vi "HStest.vi"() -> ()   [LabVIEW 2018]
uses:
  LibTiePie.lvlib
panel:
  out "Stopped?":bool
  in  "ChannelCluster":T1 {"Range" items=["0.2 Vpp"=0.2, "0.4 Vpp"=0.4, "0.8 Vpp"=0.8, "2 Vpp"=2.0, "4 Vpp"=4.0, "8 Vpp"=8.0, "20 Vpp"=20.0, "80 Vpp"=80.0]}
  out "Actual settings":T2
  in  "Settings cluster":T3={"u64RecordLength"=10000, "dPreSampleRatio"=0.2, "dSampleFrequency"=1000000.0, "MeasureMode"=2, "Bitness"=14} {"MeasureMode" items=["Block"=2, "Stream"=1]; "Bitness" items=["16 bit"=16, "14 bit"=14, "12 bit"=12]}
  out "Oscilloscoper cluster":T4
  out "Waveform Chart":dbl[][](graph)
  out "Data Out":dbl[][](array[numeric])
  out "Channel info":T5
  out "Error out":errorcluster
  out "ID out":u32
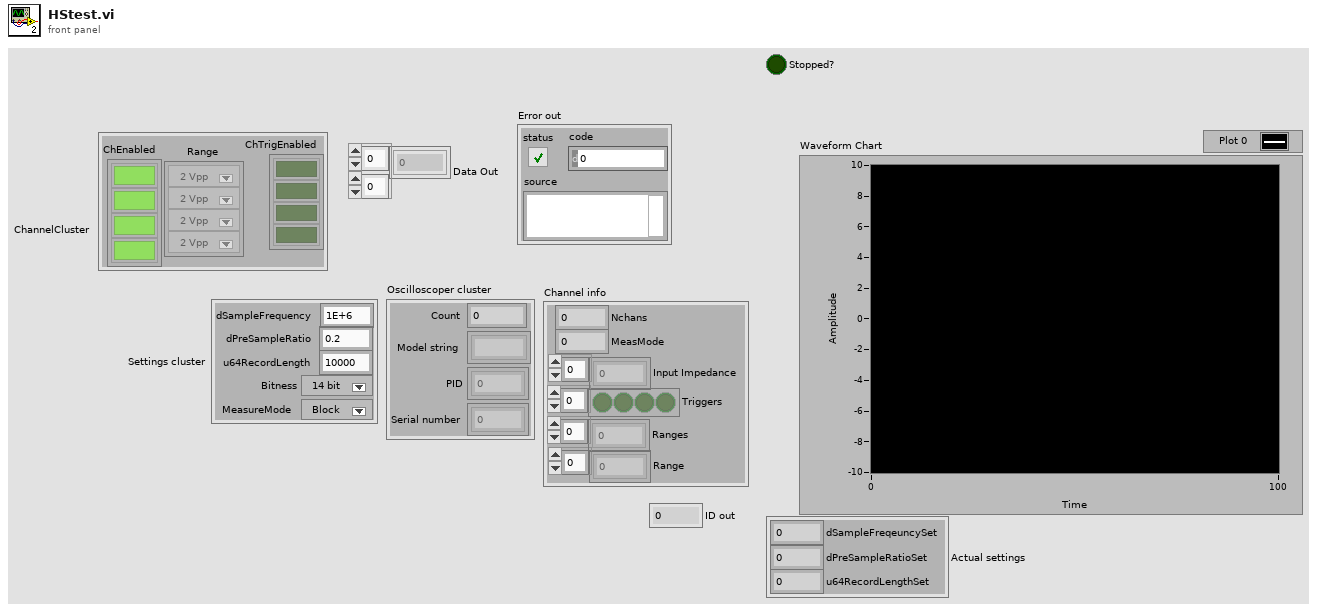
[diagram p1: front panel]
types:
  T1 = cluster{"ChEnabled":bool[], "Range":dbl[], "ChTrigEnabled":bool[]}
  T2 = cluster{"u64RecordLengthSet":u64, "dPreSampleRatioSet":dbl, "dSampleFreqeuncySet":dbl}
  T3 = cluster{"u64RecordLength":u64, "dPreSampleRatio":dbl, "dSampleFrequency":dbl, "MeasureMode":u32, "Bitness":u8}
  T4 = cluster{"Count":u32, "Model string":string[], "PID":u32[], "Serial number":u32[]}
  T5 = cluster{"Nchans":u16, "MeasMode":u32, "Input Impedance":dbl[], "Triggers":bool[], "Ranges":u32[], "Range":dbl[]}
  T6 = cluster{"Nchans":u16, "MeasMode":u32, dbl[], "Boolean array":bool[], u32[], dbl[]}
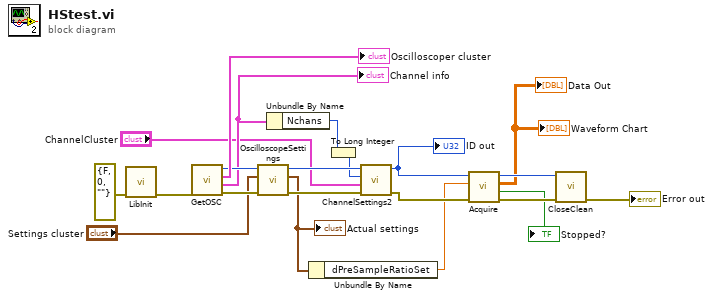
[diagram p0: block diagram]
diagram:
  n1 = call "LibInit.vi"("error in (no error)"=errorcluster {"status"=FALSE, "code"=0, "source"=""} ("error in")) -> ("error out"=w17:errorcluster)  [unwired: 10 in]
  n2 = call "GetOSC.vi"("error in"=w17) -> ("Error out"=w13:errorcluster, "Channel info"=w9:T6, "Oscilloscoper cluster"=→"Oscilloscoper cluster":T4, "Scope out"=w14:u32)  [unwired: 7 in]
  "Channel info" <- w9
  n3 = call "OscilloscopeSettings.vi"("error in (no error)"=w13, "Settings cluster"="Settings cluster", "hDevice in"=w14) -> ("error out"=w10:errorcluster, "Actual settings"=w5:T2, "hDevice out"=w11:u32)  [unwired: 6 in]
  "Actual settings" <- w5
  n4 = Unbundle By Name(w9) -> ("Nchans"=w8:u16)
  n5 = Unbundle By Name(w5) -> ("dPreSampleRatioSet"=w4:dbl)
  n6 = To Long Integer(number=w8) -> (32bit integer=w2:i32)
  n7 = call "ChannelSettings2.vi"("error in (no error)"=w10, "ChannelCluster"="ChannelCluster", "NChans"=w2, "hDevice in"=w11) -> ("error out"=w6:errorcluster, "hDevice out"=w1:u32)  [unwired: 6 in]
  "ID out" <- w1
  n8 = call "Acquire.vi"("error in (no error)"=w6, "presamp"=w4, "hDevice in"=w1) -> ("error out"=w20:errorcluster, "Stopped?"=→"Stopped?":bool, "Data Out"=→"Data Out" →"Waveform Chart":dbl[][], "hDevice out"=w19:u32)  [unwired: 5 in]
  n9 = call "CloseClean.vi"("error in (no error)"=w20, "hHandle"=w19) -> ("error out"=→"Error out":errorcluster)  [unwired: 9 in]
